vi "test save Control Values to file.vi"() -> ()   [LabVIEW 2009]
panel:
  out "file path out":path
  out "error out":errorcluster
  in  "Numeric":dbl
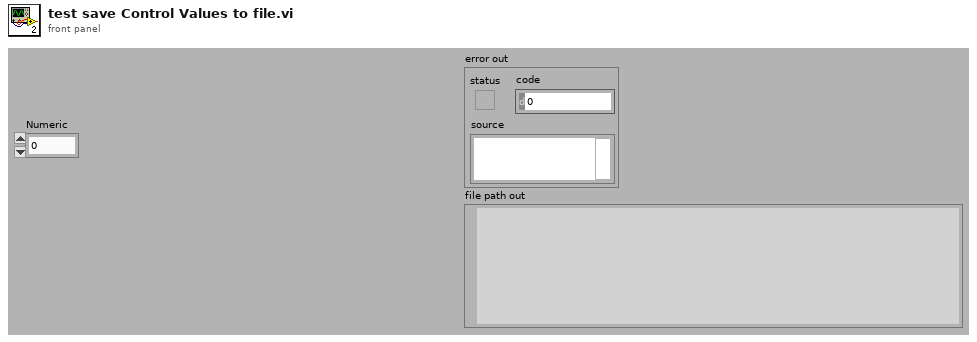
[diagram p1: front panel]
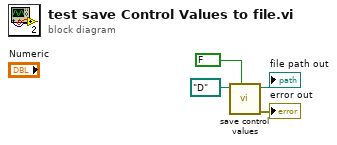
[diagram p0: block diagram]
diagram:
  n1 = call "save control values.vi"("Append timestamp (true)"=FALSE, "Path"=path "D:/") -> ("error out"=→"error out":errorcluster, "file path out"=→"file path out":path)  [unwired: 6 in]
